vi "Pre Launch Init.vi"(11 "EMS Generic in":refnum<class "EMS Generic.lvclass">) -> (0 "error out":errorcluster, 3 "EMS Generic out":refnum<class "EMS Generic.lvclass">)   [LabVIEW 2018, in "EMS Generic Actor.lvlib" / "EMS Generic.lvclass"]
doc: "(<B>Filename</B>: Actor Framework.lvlib:Actor.lvclass:Pre Launch Init.vi)\n\nDefines behavior that occurs after the Launch Nested Actor method is invoked but before the actor's Actor Core method begins running.\n\nBy default, this method does nothing. A descendant class may override it to define behavior."
uses:
  EMS Generic.lvclass
  Controls/EMS Generic Notifiers.ctl
  Controls/EMS Generic User Events.ctl
  EMS Generic.lvclass/EMS Generic.ctl
  <vilib>/ActorFramework/Actor/Actor.lvclass
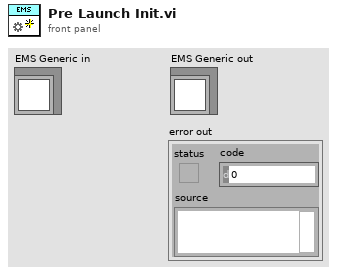
[diagram p1: front panel]
types:
  T1 = typedef "EMS Generic Actor.lvlib/EMS Generic.lvclass/EMS Generic Notifiers.ctl" = cluster{"stop":refnum<notifier>}
  T2 = typedef "EMS Generic Actor.lvlib/EMS Generic.lvclass/EMS Generic User Events.ctl" = cluster{"stop":refnum<user-event>}
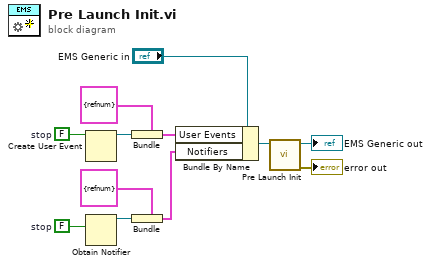
[diagram p0: block diagram]
diagram:
  w3 = FALSE  # stop
  w7 = FALSE  # stop
  n1 = Create User Event(user event datatype=w7) -> (user event=w9:refnum<user-event>)  [unwired: 1 in, 1 out]
  n2 = Obtain Notifier(notification data type=w3) -> (notifier out=w4:refnum<notifier>)  [unwired: 3 in, 2 out]
  n3 = Bundle(cluster=T2 {"stop"=refnum} ("user events"), "stop"=w9) -> (w10:T2)
  n4 = Bundle(cluster=T1 {"stop"=refnum} ("Smart Relay Notifiers"), "stop"=w4) -> (w1:T1)
  n5 = Bundle By Name(cluster="EMS Generic in", "User Events"=w10, "Notifiers"=w1) -> (w5:refnum<class "EMS Generic.lvclass">)
  n6 = call-parent "Pre Launch Init.vi"("Actor in"=w5) -> ("error out"=→"error out":errorcluster, "Actor out"=→"EMS Generic out":refnum<class "EMS Generic.lvclass">)  [unwired: 9 in]
